vi "DrawZones.vi"(8 "error in (no error)":errorcluster, 10 "Cell Size":i32, 11 "Sudoku.lvclass":refnum<class "Sudoku.lvclass">) -> (0 "error out":errorcluster, 3 "Sudoku.lvclass out":refnum<class "Sudoku.lvclass">)   [LabVIEW 2021, in "Sudoku.lvclass"]
uses:
  Sudoku.lvclass
  Sudoku.lvclass/Sudoku.ctl
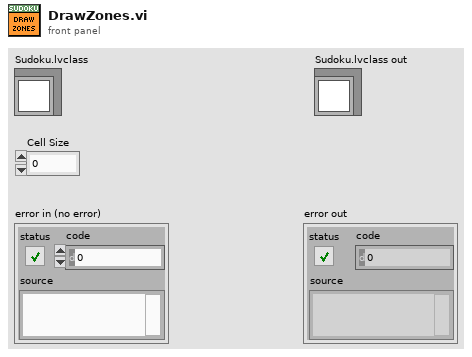
[diagram p1: front panel]
types:
  T1 = cluster{"left":i16, "top":i16, "right":i16, "bottom":i16}
  T2 = cluster{"Width":i16, "Style":enum32{"Solid", "Dash", "Dot", "DashDot", "DashDotDot"}}
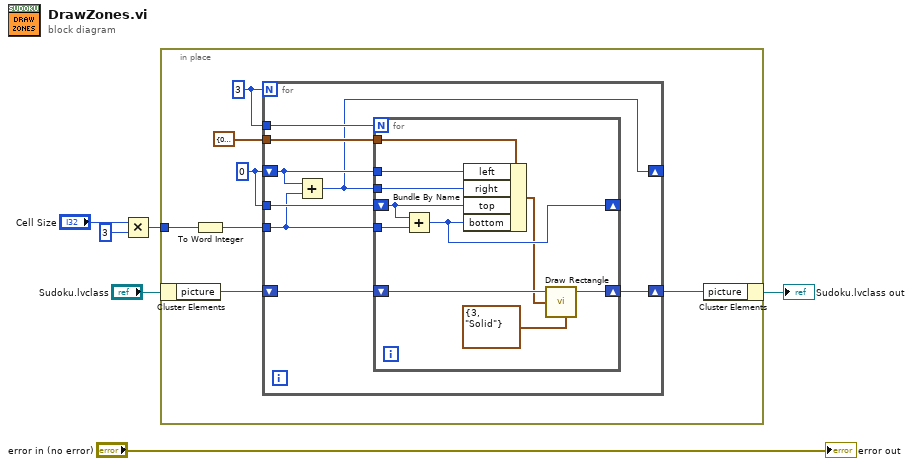
[diagram p0: block diagram]
diagram:
  n1 = Multiply(x="Cell Size", y=3) -> (x*y=w2:i32)
  n2 = in-place {
    in-place-border: w2 -> [w9]
    w7 = i16 0 ("left")
    w10 = 3
    n3 = in-place-cluster #1("Sudoku.lvclass") -> ("picture"=w13:picture)
    n4 = To Word Integer(number=w9) -> (16bit integer=w8:i16)
    n5 = for {
      N: w10 -> [_]
      shift-right: [w20] -> w12
      shift-left: w13 -> [w21]
      tunnel: T1 {"left"=0, "top"=0, "right"=0, "bottom"=0} ("rect") -> [w19]
      tunnel: w10 -> [w18]
      shift-right: [w16] -> _
      shift-left: w7 -> [w17]
      tunnel: w8 -> [w14]
      tunnel: w7 -> [w15]
      n6 = Add(x=w17, y=w14) -> (x+y=w16:i16)
      n7 = for {
        N: w18 -> [_]
        shift-right: [w30] -> w20
        shift-left: w21 -> [w31]
        tunnel: w19 -> [w29]
        tunnel: w17 -> [w28]
        tunnel: w16 -> [w27]
        shift-right: [w25] -> _
        shift-left: w15 -> [w26]
        tunnel: w14 -> [w24]
        n8 = Add(x=w26, y=w24) -> (x+y=w25:i16)
        n9 = Bundle By Name(cluster=w29, "left"=w28, "right"=w27, "top"=w26, "bottom"=w25) -> (w23:T1)
        n10 = call <vilib>:"Draw Rectangle.vi"("picture"=w31, "rect"=w23, "pen"=T2 {"Width"=3, "Style"=enum."Solid"}) -> ("new picture"=w30:picture)  [unwired: 6 in]
      }
    }
    n11 = in-place-cluster #1("picture"=w12) -> (→"Sudoku.lvclass out":refnum<class "Sudoku.lvclass">)
  }
  "error out" <- "error in (no error)"
